vi "I2C Generator.vi"(5 "I2C Generator Fgen Channel":string, 6 "duration":dbl, 7 "I2C waveform":T1, 8 "error in (no error)":errorcluster, 9 "I2C amplitude":dbl, 10 "I2C frequency":dbl, 11 "IVI Refnum in":refnum<k15>) -> (0 "error out":errorcluster, 3 "Numeric":dbl)   [LabVIEW 2021, in "Waveform Generator T1.lvlib"]
uses:
  Waveform Generator T1.lvlib
  controls/Type.ctl
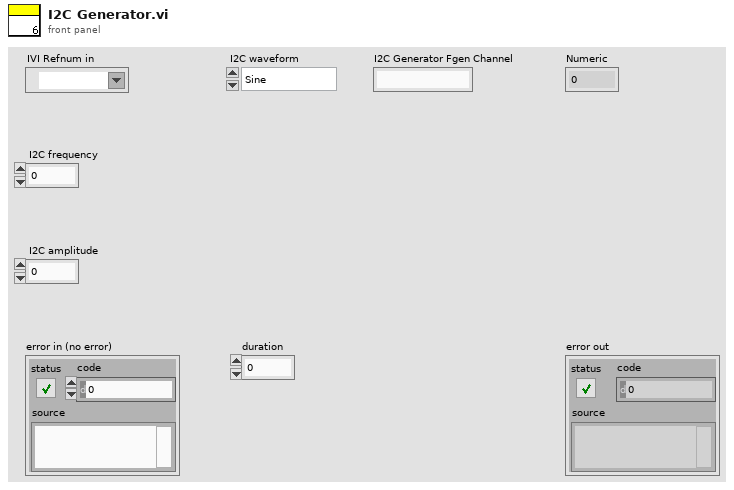
[diagram p1: front panel]
types:
  T1 = typedef "Waveform Generator T1.lvlib/Type.ctl" = enum32{"Sine", "Square", "Triangle", "Ramp Up", "Ramp Down", "DC", "Noise", "User"}
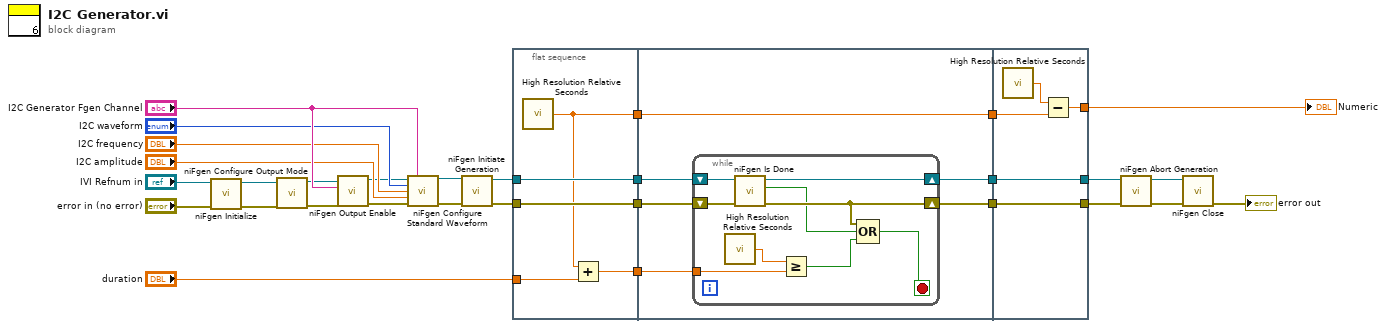
[diagram p0: block diagram]
diagram:
  n1 = call <instrlib>:"niFgen Initialize.vi"("error in (no error)"="error in (no error)", "Resource Name"="IVI Refnum in") -> ("error out"=w4:errorcluster, "Instrument Handle Out"=w1:refnum<k15>)  [unwired: 8 in]
  n2 = call <instrlib>:"niFgen Configure Output Mode.vi"("error in (no error)"=w4, "Instrument Handle"=w1) -> ("error out"=w15:errorcluster, "Instrument Handle Out"=w5:refnum<k15>)  [unwired: 7 in]
  n3 = call <instrlib>:"niFgen Output Enable.vi"("error in (no error)"=w15, "Channel Name"="I2C Generator Fgen Channel", "Instrument Handle"=w5) -> ("error out"=w3:errorcluster, "Instrument Handle Out"=w6:refnum<k15>)  [unwired: 7 in]
  n4 = call <instrlib>:"niFgen Configure Standard Waveform.vi"("Instrument Handle"=w6, "Channel Name"="I2C Generator Fgen Channel", "Waveform"="I2C waveform", "Frequency"="I2C frequency", "Amplitude"="I2C amplitude", "error in (no error)"=w3) -> ("Instrument Handle Out"=w7:refnum<k15>, "error out"=w2:errorcluster)  [unwired: 8 in]
  n5 = call <instrlib>:"niFgen Initiate Generation.vi"("error in (no error)"=w2, "Instrument Handle"=w7) -> ("error out"=w10:errorcluster, "Instrument Handle Out"=w8:refnum<k15>)  [unwired: 8 in]
  n6 = flat-sequence {
    tunnel: w10 -> [w34]
    tunnel: w8 -> [w35]
    tunnel: [w35] -> w30
    tunnel: [w34] -> w29
    tunnel: [w33] -> w28
    tunnel: "duration" -> [w32]
    tunnel: [w31] -> w27
    tunnel: w30 -> [w41]
    tunnel: w29 -> [w39]
    tunnel: [w40] -> w26
    tunnel: [w38] -> w25
    tunnel: [w37] -> w24
    tunnel: w28 -> [w37]
    tunnel: w27 -> [w36]
    tunnel: [w54] -> w11
    tunnel: [w55] -> w9
    tunnel: w26 -> [w55]
    tunnel: w25 -> [w54]
    tunnel: w24 -> [w52]
    tunnel: [w51] -> w21
    frame #0 {
      n7 = call <vilib>:"High Resolution Relative Seconds.vi"() -> ("relative seconds"=w33:dbl)
      n8 = Add(x=w33, y=w32) -> (x+y=w31:dbl)
    }
    frame #1 {
      n9 = while {
        shift-right: [w49] -> w40
        shift-left: w41 -> [w50]
        shift-right: [w47] -> w38
        shift-left: w39 -> [w48]
        tunnel: w36 -> [w44]
        stop <- w46 stop-if-true
        n10 = call <vilib>:"High Resolution Relative Seconds.vi"() -> ("relative seconds"=w45:dbl)
        n11 = call <instrlib>:"niFgen Is Done.vi"("error in (no error)"=w48, "Instrument Handle"=w50) -> ("error out"=w47:errorcluster, "Done"=w42:bool, "Instrument Handle Out"=w49:refnum<k15>)  [unwired: 7 in]
        n12 = Greater Or Equal?(x=w45, y=w44) -> (x >= y?=w43:bool)
        n13 = Compound Arithmetic op=OR(w47, w42, w43) -> (w46:bool)
      }
    }
    frame #2 {
      n14 = call <vilib>:"High Resolution Relative Seconds.vi"() -> ("relative seconds"=w53:dbl)
      n15 = Subtract(x=w53, y=w52) -> (x-y=w51:dbl)
    }
  }
  n16 = call <instrlib>:"niFgen Abort Generation.vi"("error in (no error)"=w11, "Instrument Handle"=w9) -> ("error out"=w13:errorcluster, "Instrument Handle Out"=w12:refnum<k15>)  [unwired: 8 in]
  n17 = call <instrlib>:"niFgen Close.vi"("error in (no error)"=w13, "Instrument Handle"=w12) -> ("error out"=→"error out":errorcluster)  [unwired: 9 in]
  "Numeric" <- w21
